vi "Test App Set and Get Process.vi"(8 "error in (no error)":errorcluster, 11 "Application Test in":refnum<class "Application Test.lvclass">) -> (0 "error out":errorcluster, 3 "Application Test out":refnum<class "Application Test.lvclass">)   [LabVIEW 2020, in "Application Test.lvclass"]
uses:
  Application Test.lvclass
  C:/Program Files (x86)/National Instruments/LabVIEW 2020/vi.lib/Asteme/LUnit/Test Case.lvclass
  Framework/Process/Process.lvclass
  Framework/Process/Process.lvclass/Process.ctl
  Framework/Application/Application.lvclass/Application.ctl
  <vilib>/Asteme/LUnit/Test Case.lvclass/Test Case.ctl
  <vilib>/Asteme/LUnit/LUnit Assertion Result.lvclass/LUnit Assertion Result.ctl
  Framework/Process/Protected/SubVIs/Set Context.vi
  Framework/Application/Private/Add Process to Map.vi
  Framework/Process/Protected/Messaging/Enqueue Message.vi
  Framework/Process/Public/Get Lifecycle State.vi
  Framework/Process/Protected/Messaging/Request Message.vi
  Framework/Process/Protected/SubVIs/Get Access Mode.vi
  <vilib>/Asteme/LUnit/Palette/Fail.vi
  <vilib>/Asteme/LUnit/Palette/Pass.vi
  <vilib>/Asteme/LUnit/Set Assertion Type.vi
  Framework/Process/Private/SubVIs/Wait for finish.vi
  Framework/Process/Private/SubVIs/Set Lifecycle State.vi
  <vilib>/AdvancedString/1D String Array to Delimited String.vi
  <vilib>/Utility/error.llb/Clear Errors.vi
  Framework/Process/Private/SubVIs/Enqueue Request Message.vi
  <vilib>/Asteme/LUnit/Add test result.vi
  <vilib>/Asteme/LUnit/LUnit Write Passed.vi
  <vilib>/Asteme/LUnit/LUnit Get Test Case.vi
  <vilib>/Asteme/LUnit/LUnit Write Message.vi
  <vilib>/Asteme/LUnit/LUnit Write Description.vi
  <vilib>/Asteme/LUnit/LUnit Write Assertion Type.vi
  <vilib>/Asteme/LUnit/Read Test Case Name.vi
  Framework/Application/Application.lvclass
  C:/Users/anton/Documents/GitHub/Triarc-Framework/source/Framework/Process/Process.lvclass
  <vilib>/Utility/error.llb/Error Cluster From Error Code.vi
  Framework/Process/Private/SubVIs/Wait for Response Message.vi
  <vilib>/Asteme/LUnit/Assertion Result/LUnit Get Test Name.vi
  <vilib>/Asteme/LUnit/LUnit Assertion Result.lvclass
  <vilib>/Asteme/LUnit/Test Case.lvclass
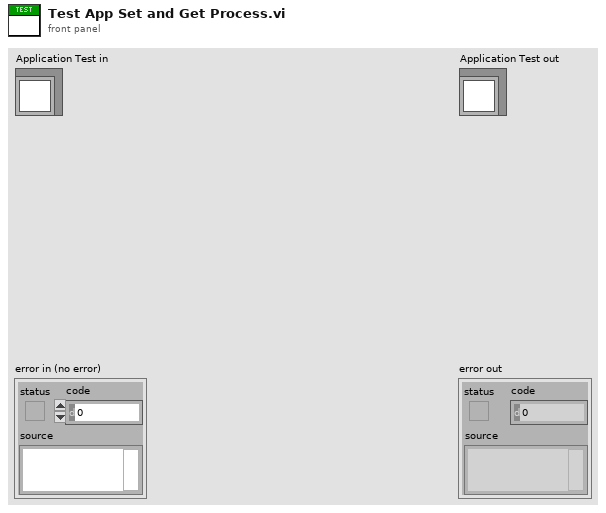
[diagram p1: front panel]
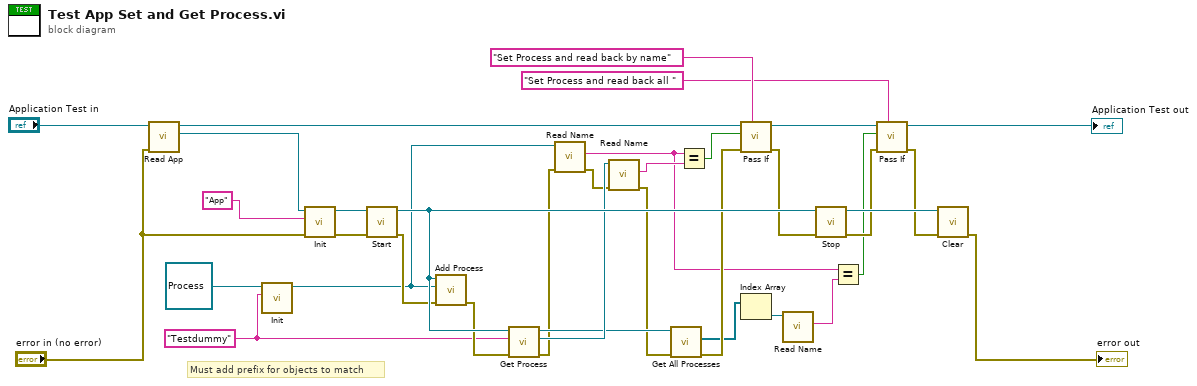
[diagram p0: block diagram]
diagram:
  w11 = "Testdummy" ("Name")
  # "Must add prefix for objects to match"
  n1 = call "Read App.vi"("error in (no error)"="error in (no error)", "Application Test In"="Application Test in") -> ("App out"=w34:refnum<class "Application.lvclass">, "Application Test Out"=w35:refnum<class "Application Test.lvclass">)  [unwired: 7 in, 1 out]
  n2 = call-dynamic "Init.vi"("Name"=w11, "Process In"=refnum<class "Process.lvclass"> refnum ("Process.lvclass")) -> ("Process Out"=w6:refnum<class "Process.lvclass">)  [unwired: 8 in, 1 out]
  n3 = call-dynamic "Init.vi"("error in (no error)"="error in (no error)", "Name"="App", "Process In"=w34) -> ("error out"=w32:errorcluster, "Process Out"=w33:refnum<class "Application.lvclass">)  [unwired: 7 in]
  n4 = call "Start.vi"("error in (no error)"=w32, "Process In"=w33) -> ("error out"=w28:errorcluster, "Process Out"=w30:refnum<class "Application.lvclass">)  [unwired: 8 in]
  n5 = call "Add Process.vi"("error in (no error)"=w28, "Process"=w6, "Rig In"=w30) -> ("error out"=w29:errorcluster)  [unwired: 7 in, 1 out]
  n6 = call "Get Process.vi"("error in (no error)"=w29, "Process Name"=w11, "Rig In"=w30) -> ("error out"=w2:errorcluster, "App Process"=w25:refnum<class "Process.lvclass">, "Rig Out"=w21:refnum<class "Application.lvclass">)  [unwired: 6 in]
  n7 = call-dynamic "Read Name.vi"("error in (no error)"=w2, "Process In"=w6) -> ("error out"=w3:errorcluster, "Qualified Name"=w5:string)  [unwired: 6 in, 2 out]
  n8 = call-dynamic "Read Name.vi"("error in (no error)"=w3, "Process In"=w25) -> ("error out"=w1:errorcluster, "Qualified Name"=w7:string)  [unwired: 6 in, 2 out]
  n9 = call "Get All Processes.vi"("error in (no error)"=w1, "Application In"=w21) -> ("error out"=w23:errorcluster, "App Processes"=w20:refnum<class "Process.lvclass">[])  [unwired: 7 in, 1 out]
  n10 = Equal?(x=w5, y=w7) -> (x = y?=w24:bool)
  n11 = call <vilib>:"Pass If.vi"("Description"="Set Process and read back by name", "error in (no error)"=w23, "Pass?"=w24, "Test Case In"=w35) -> ("error out"=w22:errorcluster, "Test Case Out"=w26:refnum<class "Application Test.lvclass">)  [unwired: 6 in]
  n12 = Index Array(array=w20) -> (element=w19:refnum<class "Process.lvclass">)  [unwired: 1 in]
  n13 = call-dynamic "Read Name.vi"("Process In"=w19) -> ("Qualified Name"=w4:string)  [unwired: 7 in, 3 out]
  n14 = call "Stop.vi"("error in (no error)"=w22, "Process In"=w30) -> ("error out"=w15:errorcluster, "Process Out"=w31:refnum<class "Application.lvclass">)  [unwired: 7 in, 1 out]
  n15 = Equal?(x=w5, y=w4) -> (x = y?=w13:bool)
  n16 = call <vilib>:"Pass If.vi"("Description"="Set Process and read back all ", "error in (no error)"=w15, "Pass?"=w13, "Test Case In"=w26) -> ("error out"=w14:errorcluster, "Test Case Out"=→"Application Test out":refnum<class "Application Test.lvclass">)  [unwired: 6 in]
  n17 = call-dynamic "Clear.vi"("error in (no error)"=w14, "Application In"=w31) -> ("error out"=→"error out":errorcluster)  [unwired: 8 in, 1 out]
